vi "dlw_TCP Client.vi"(6 "Worker Alias":string="TCP Client", 7 "Caller in":refnum<class "Worker.lvclass">, 8 "error in":errorcluster, 10 "Initialization Data":T1, 11 "TCP Client in":refnum<class "TCP Client.lvclass">) -> (0 "error out":errorcluster, 3 "TCP Client out":refnum<class "TCP Client.lvclass">, 5 "dup Caller out":refnum<class "Worker.lvclass">)   [LabVIEW 2017, in "TCP Client.lvlib" / "TCP Client.lvclass"]
doc: "This VI dynamically loads the Worker that owns this VI as a subWorker into <b>Caller</b>, and returns the Worker's object containing the Worker's Public Properties. Initialization data that is to be received by this Worker's <Initialize> MHL case can be wired to <b>Initialization Data</b>. The dynamically loaded Worker requires an alias ( <b>Worker Alias</b> ) which must be unique to the Worker it is called from. If a currently loaded subWorker exists with the same Alias, an error will be returned.\n\n<b>Note:</b> This VI can only be called from <b>within</b> another Worker. To call this Worker from an external LabVIEW application, load this Worker with an Asynchronous Launcher VI.\n---"
uses:
  TCP Client.lvclass
  C:/Program Files (x86)/National Instruments/LabVIEW 2017/vi.lib/addons/_Workers/Library/Classes/Worker/Worker.lvclass
  <vilib>/addons/_Workers/Library/Classes/Worker/Worker.lvclass
  Initialization Data.ctl
  Response Cases.ctl
  <vilib>/addons/_Workers/Library/Case Label.ctl
  <vilib>/addons/_Workers/Library/Workers.lvlib
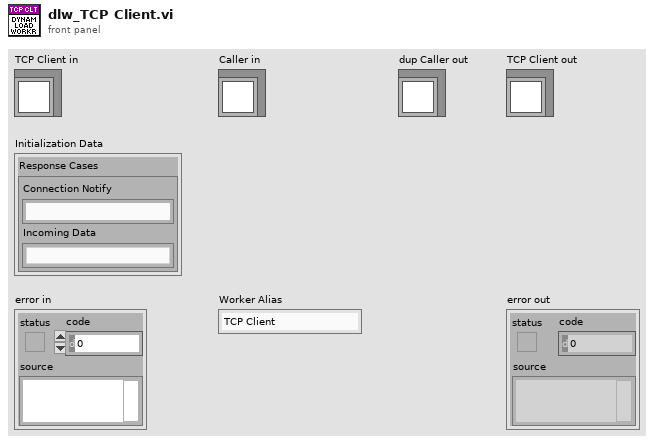
[diagram p1: front panel]
types:
  T1 = typedef "TCP Client.lvlib/TCP Client.lvclass/Initialization Data.ctl" = cluster{"Response Cases":T2}
  T2 = typedef "TCP Client.lvlib/TCP Client.lvclass/Response Cases.ctl" = cluster{"Connection Notify":T3, "Incoming Data":T3}
  T3 = typedef "Workers.lvlib/Case Label.ctl" = string
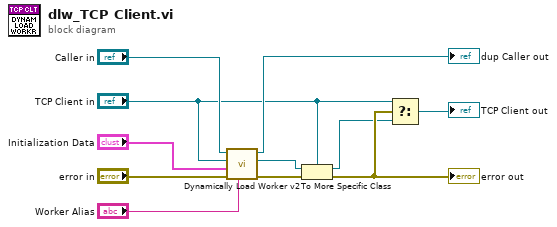
[diagram p0: block diagram]
diagram:
  n1 = call <vilib>:"Dynamically Load Worker v2.vi"("Worker Alias"="Worker Alias", "error in"="error in", "Initialization Data"="Initialization Data", "Worker to Dynamically Load"="TCP Client in", "Worker"="Caller in") -> ("error out"=w10:errorcluster, "Dynamically Loaded Worker out"=w5:refnum<class "Worker.lvclass">, "dup Worker out"=→"dup Caller out":refnum<class "Worker.lvclass">)  [unwired: 4 in]
  n2 = To More Specific Class(target class="TCP Client in", reference=w5, error in=w10) -> (specific class reference=w2:refnum<class "TCP Client.lvclass">, error out=w4:errorcluster)
  "error out" <- w4
  n3 = Select(t="TCP Client in", s=w4, f=w2) -> (s? t:f=→"TCP Client out":refnum<class "TCP Client.lvclass">)
